vi "Read IT.vi"(10 "IT":i32, 11 "handle":i32) -> (1 "function return":i32, 2 "IT out":i32, 3 "handle out":i32)   [LabVIEW 2022 SP3]
doc: "BOOL H11890API __stdcall H11890ReadIT(HANDLE handle,DWORD *IT);"
uses:
  H11890api.dll
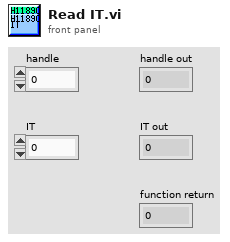
[diagram p1: front panel]
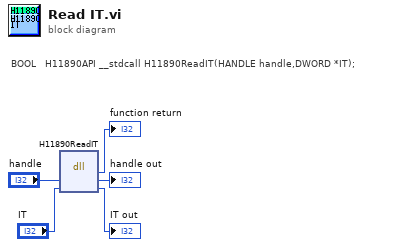
[diagram p0: block diagram]
diagram:
  # "BOOL\t\t\tH11890API\t__stdcall H11890ReadIT(HANDLE handle,DWORD *IT);"
  n1 = dll-call lib="C:/Users/Public/OneDrive/Desktop/PMT_Project_folder/PMT_VIs/H11890api.dll" fn="H11890ReadIT"("handle"="handle", "IT"="IT") -> ("Return"=→"function return":i32, "handle"=→"handle out":i32, "IT"=→"IT out":i32)  [unwired: 3 in, 2 out]
